vi "p1.vi"() -> ()   [LabVIEW 2025, in "d2.lvlib"]
uses:
  d2.lvlib
  lv2025-aoc/AOC/AOC.lvlib
panel:
  in  "Example":string="11-22,95-115,998-1012,1188511880-1188511890,222220-222224,\n1698522-1698528,446443-446449,38593856-38593862,565653-565659,\n824824821-824824827,2121212118-2121212124"
  in  "Example":bool
  out "Answer":i64=10624
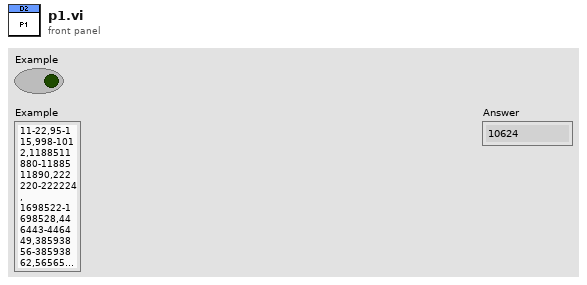
[diagram p1: front panel]
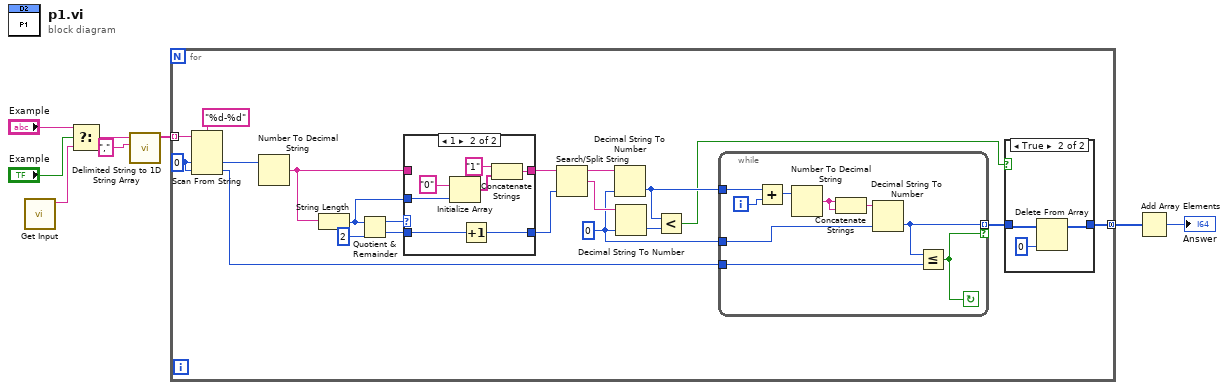
[diagram p0: block diagram]
diagram:
  n1 = call "Get Input.vi"() -> ("Input"=w8:string)  [unwired: 11 in]
  n2 = Select(t="Example", s="Example", f=w8) -> (s? t:f=w7:string)
  n3 = call <vilib>:"Delimited String to 1D String Array.vi"("delimiter"=",", "delimited string"=w7) -> ("string array"=w5:string[])  [unwired: 9 in]
  n4 = for {
    tunnel: w5 -> [w28] mode=indexing
    tunnel: [w13] -> w2 mode=concatenating
    w11 = i64 0 ("default value 14")
    w12 = i64 0 ("default (0 I32)")
    n5 = Scan From String(format string="%d-%d", input string=w28, default 1=w11, default 2=w11) -> (output 1=w26:i64, output 2=w24:i64)  [unwired: 2 in, 3 out]
    n6 = Number To Decimal String(number=w26) -> (decimal integer string=w17:string)  [unwired: 1 in]
    n7 = String Length(string=w17) -> (length=w15:i32)
    n8 = Quotient & Remainder(x=w15, y=2) -> (x-y*floor(x/y)=w18:i32, floor(x/y)=w10:i32)
    n9 = case shown="1" w18 {
      tunnel: w17 -> [w30 _]
      tunnel: [w30 w35] -> w16
      tunnel: w15 -> [_ w37]
      tunnel: w10 -> [w29 w32]
      tunnel: [w29 w31] -> w9
      frame 0, Default {
      }
      frame 1 {
        n10 = Initialize Array("0" ("format string"), w37) -> (w34:string[])
        n11 = Increment(x=w32) -> (x+1=w31:i32)
        n12 = Concatenate Strings("1" ("string"), w34) -> (w35:string)
      }
    }
    n13 = Search/Split String(string=w16, offset (0)=w9) -> (substring before match=w23:string, match + rest of string=w22:string)  [unwired: 1 in, 1 out]
    n14 = Decimal String To Number(string=w23, default (0L)=w12) -> (number=w20:i64)  [unwired: 1 in, 1 out]
    n15 = Decimal String To Number(string=w22, default (0L)=w12) -> (number=w21:i64)  [unwired: 1 in, 1 out]
    n16 = Less?(x=w20, y=w21) -> (x < y?=w19:bool)
    n17 = while {
      tunnel: w20 -> [w46]
      tunnel: w24 -> [w43]
      tunnel: [w40] -> w14 mode=indexing if=w39
      tunnel: w12 -> [w38]
      i -> [w41]
      stop <- w39 continue-if-true
      n18 = Add(x=w46, y=w41) -> (x+y=w45:i64)
      n19 = Number To Decimal String(number=w45) -> (decimal integer string=w44:string)  [unwired: 1 in]
      n20 = Concatenate Strings(w44, w44) -> (w42:string)
      n21 = Decimal String To Number(string=w42, default (0L)=w38) -> (number=w40:i64)  [unwired: 1 in, 1 out]
      n22 = Less Or Equal?(x=w40, y=w43) -> (x <= y?=w39:bool)
    }
    n23 = case shown="True" w19 {
      tunnel: w14 -> [w47 w50]
      tunnel: [w47 w49] -> w13
      frame False {
      }
      frame True {
        n24 = Delete From Array(array=w50, index=0) -> (array with subset deleted=w49:i64[])  [unwired: 1 in, 1 out]
      }
    }
  }
  n25 = Add Array Elements(numeric array=w2) -> (sum=→"Answer":i64)
